vi "Cerrar.vi"(8 "error in (no error)":errorcluster, 11 "Camara in":refnum<class "Camara.lvclass">) -> (0 "error out":errorcluster, 3 "Camara out":refnum<class "Camara.lvclass">)   [LabVIEW 2020, in "Camara.lvclass"]
uses:
  Camara.lvclass
  Camara.lvclass/Camara.ctl
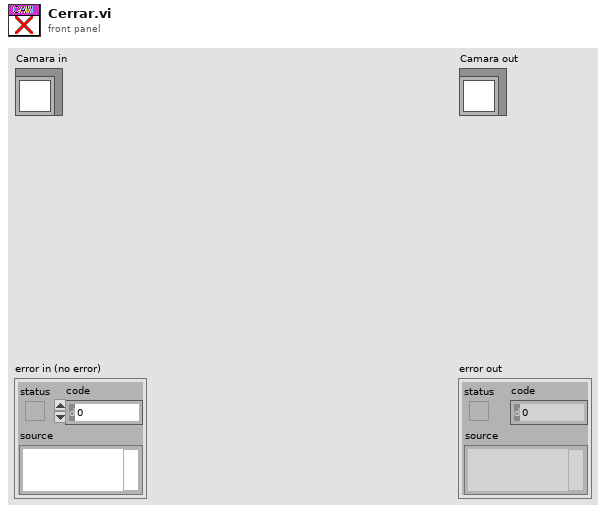
[diagram p1: front panel]
types:
  T1 = typedef "IMAQ Image.ctl" = refnum<image>
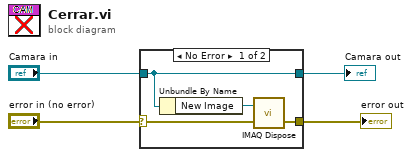
[diagram p0: block diagram]
diagram:
  n1 = case shown="No Error" "error in (no error)" {
    selector: "error in (no error)" -> [w6 w10]
    tunnel: [w5 w10] -> w3
    tunnel: [w8 w9] -> w1
    tunnel: "Camara in" -> [w8 w9]
    frame No Error {
      n2 = Unbundle By Name(w8) -> ("New Image"=w7:T1)
      n3 = call "IMAQ Dispose"("Image"=w7, "error in (no error)"=w6) -> ("error out"=w5:errorcluster)  [unwired: 4 in]
    }
    frame Error {
    }
  }
  "error out" <- w3
  "Camara out" <- w1
